vi "Finalize Hardware.vi"(6 "force (F)":bool, 8 "error in":errorcluster, 11 "boardId":u8) -> (0 "error out":errorcluster)   [LabVIEW 2020, in "AIM ARINC 429 Hardware API.lvlib"]
uses:
  AIM ARINC 429 Hardware API.lvlib
  <instrlib>/_AIM 429/Controls/HwManager_action.ctl
  <instrlib>/_AIM 429/AIM429LV.lvlib
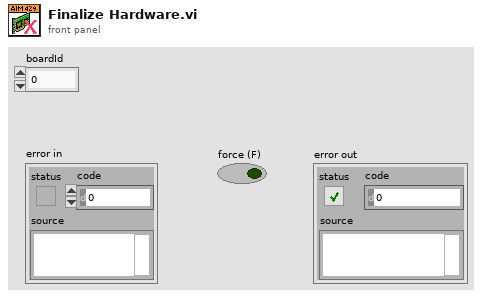
[diagram p1: front panel]
types:
  T1 = typedef "AIM429LV.lvlib/HwManager_action.ctl" = enum16{"Get Resource", "Remove Instance", "Add Resource", "Clear All", "Remove Resource"}
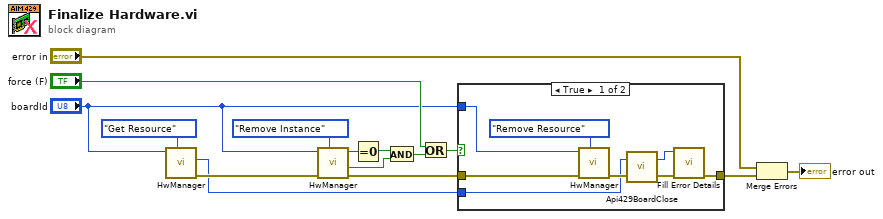
[diagram p0: block diagram]
diagram:
  n1 = call <instrlib>:"HwManager.vi"("Action (Get)"=HwManager_action."Get Resource", "board id"="boardId") -> ("error out"=w7:errorcluster, "module handle out"=w4:u8)  [unwired: 6 in, 2 out]
  n2 = call <instrlib>:"HwManager.vi"("Action (Get)"=HwManager_action."Remove Instance", "error in (no error)"=w7, "board id"="boardId") -> ("error out"=w8:errorcluster, "found"=w11:bool, "# of board instances"=w9:i32)  [unwired: 5 in, 1 out]
  n3 = Equal To 0?(x=w9) -> (x = 0?=w10:bool)
  n4 = And(x=w10, y=w11) -> (x .and. y?=w12:bool)
  n5 = Or(x="force (F)", y=w12) -> (x .or. y?=w13:bool)
  n6 = case shown="True" w13 {
    tunnel: w8 -> [w23 w24]
    tunnel: [w18 w24] -> w3
    tunnel: "boardId" -> [w21 _]
    tunnel: w4 -> [w17 _]
    frame True {
      n7 = call <instrlib>:"HwManager.vi"("Action (Get)"=HwManager_action."Remove Resource", "error in (no error)"=w23, "board id"=w21) -> ("error out"=w19:errorcluster)  [unwired: 5 in, 3 out]
      n8 = call <instrlib>:"Api429BoardClose.vi"("error in (no error)"=w19, "bmodule"=w17) -> ("error out"=w20:errorcluster, "error code"=w16:i32)
      n9 = call "Fill Error Details.vi"("error in"=w20, "error code"=w16) -> ("error out"=w18:errorcluster)  [unwired: 9 in]
    }
    frame False {
    }
  }
  n10 = Merge Errors("error in", w3) -> (→"error out":errorcluster)
